vi "ComputeFileNameFromTime.vi"(3 "File name extension":string="txt", 4 "File name base":string="test", 5 "Output directory":string="/home/operator/data") -> (0 "TIme used":timestamp, 1 "Output file path":path, 2 "Output file name":string)   [LabVIEW 2009]
doc: "Test out attenuation switching."
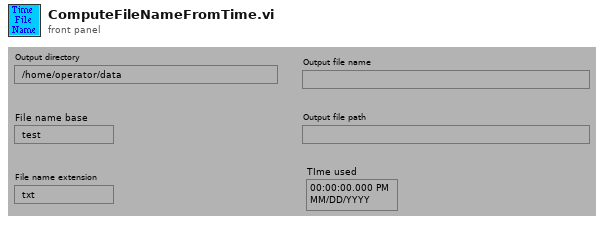
[diagram p1: front panel]
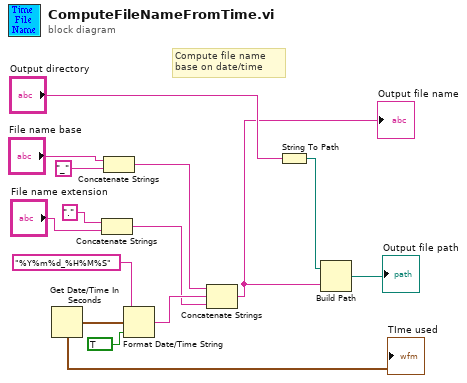
[diagram p0: block diagram]
diagram:
  # "Compute file name base on date/time"
  n1 = Get Date/Time In Seconds() -> (seconds since 1Jan1904=w7:timestamp)
  "TIme used" <- w7
  n2 = Concatenate Strings(".", "File name extension") -> (w1:string)
  n3 = Concatenate Strings("File name base", "_") -> (w2:string)
  n4 = Format Date/Time String(time format string (%c)="%Y%m%d_%H%M%S", seconds (now)=w7, UTC format=TRUE) -> (date/time string=w9:string)
  n5 = Concatenate Strings(w2, w9, w1) -> (w10:string)
  "Output file name" <- w10
  n6 = String To Path(string="Output directory") -> (path=w11:path)
  n7 = Build Path(base path=w11, name or relative path=w10) -> (appended path=→"Output file path":path)
